vi "Teleop.vi"(10 "Match Info":T1={"Autonomous Elapsed Seconds"=0.0, "TeleOp Elapsed Seconds"=0.0, "Disabled Elapsed Seconds"=0.0, "Visited Autonomous"=FALSE, "Visited TeleOp"=FALSE, "Visited Disabled"=FALSE, "Autonomous Settings"={"Autonomous Style"=enum."Independent", "VI Refnum"=refnum}}, 11 "Call Context":T2) -> ()   [LabVIEW 2017]
doc: "This VI is called for each enabled TeleOp packet received from the DS. It is typically used to read from joysticks and other inputs and update I/O or setpoints for timed control loops. It should complete and return within 20 milliseconds or risk missing DS packets."
uses:
  <vilib>/Rock Robotics/WPI/DriverStation/WPI_DriverStationDerivedRobotMode.ctl
  <vilib>/Rock Robotics/WPI/DriverStation/WPI_DriverStationMatch Info.ctl
  <vilib>/Rock Robotics/WPI/Utilities/WPI_GetSetVariantRefNum.vi
  <vilib>/Rock Robotics/Network Tables/NT Write Boolean Array.vi
  <vilib>/Rock Robotics/Network Tables/NT Write Numeric Array.vi
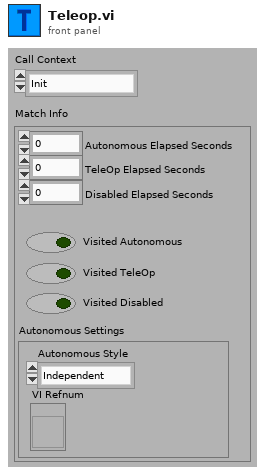
[diagram p1: front panel]
types:
  T1 = typedef "WPI_DriverStationMatch Info.ctl" = cluster{"Autonomous Elapsed Seconds":dbl, "TeleOp Elapsed Seconds":dbl, "Disabled Elapsed Seconds":dbl, "Visited Autonomous":bool, "Visited TeleOp":bool, "Visited Disabled":bool, "Autonomous Settings":cluster{"Autonomous Style":enum16{"Iterative", "Independent"}, "VI Refnum":refnum<vi>}}
  T2 = typedef "WPI_DriverStationDerivedRobotMode.ctl" = enum16{"Init", "Execute", "Stop"}
  T3 = typedef "WPI_JoystickDevRef.ctl" = cluster{"Device":T4}
  T4 = typedef "WPI_JoystickDeviceEnum.ctl" = enum16{"USB 0", "USB 1", "USB 2", "USB 3", "USB 4", "USB 5"}
  T5 = typedef "Command Status Info.ctl" = cluster{"Name":string, "Status":T6, "notifier out":T7}
  T6 = typedef "Completion Status.ctl" = enum16{"Successful", "Aborted", "Incomplete"}
  T7 = typedef "Completion Notifier.ctl" = refnum<notifier>
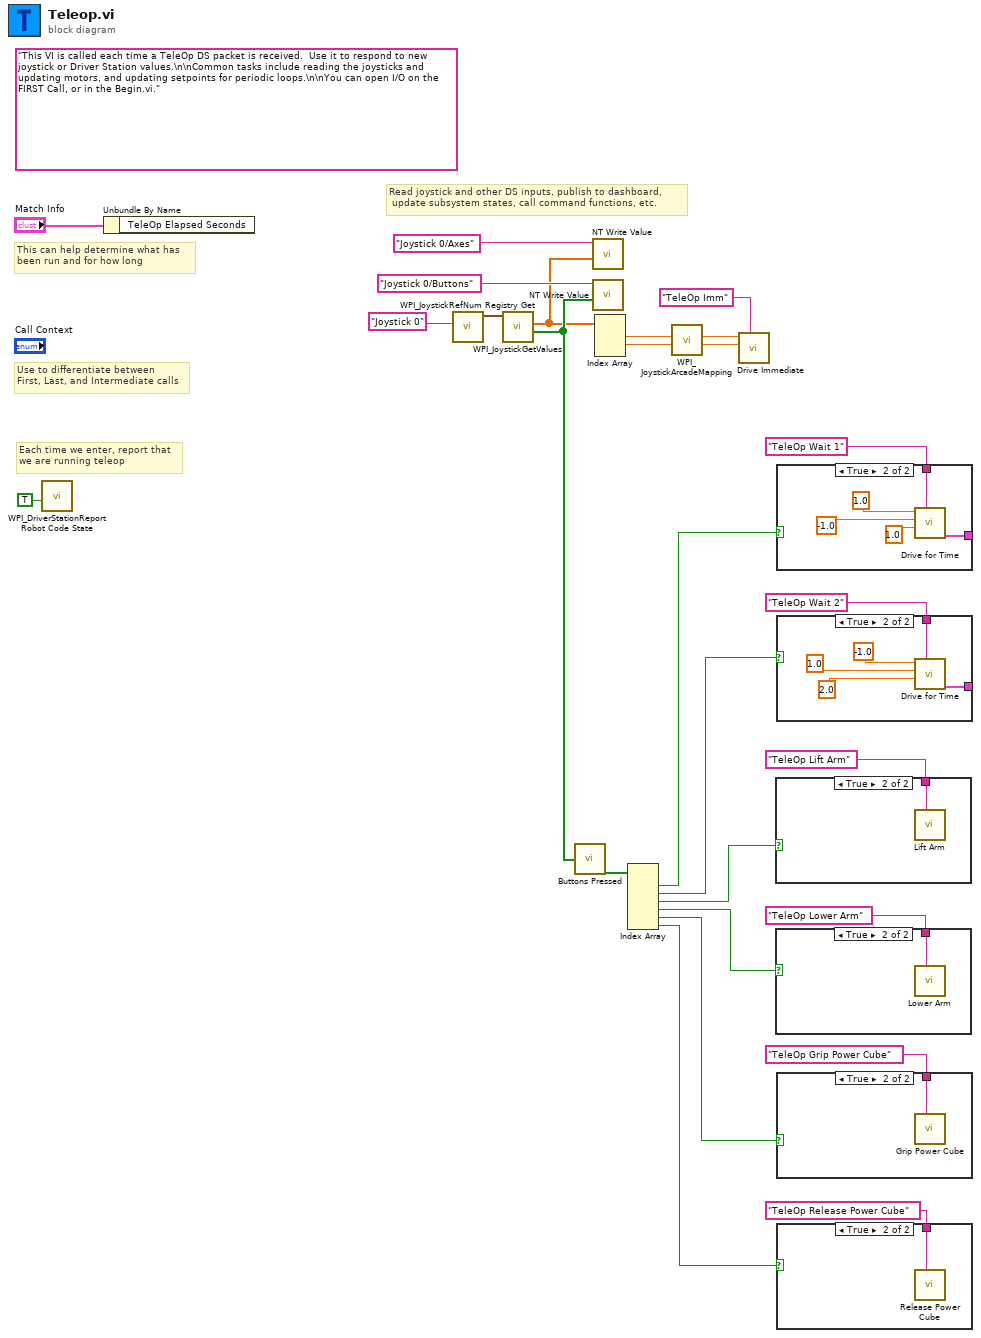
[diagram p0: block diagram]
diagram:
  (unwired) "This VI is called each time a TeleOp DS packet is received.  Use it to respond to new joystick or Driver Station values.\n\nCommon tasks include reading the joysticks and updating motors, and updating setpoints for periodic loops.\n\nYou can open I/O on the FIRST Call, or in the Begin.vi."
  # "Read joystick and other DS inputs, publish to dashboard,\n update subsystem states, call command functions, etc."
  # "Each time we enter, report that\nwe are running teleop"
  # "Use to differentiate between\nFirst, Last, and Intermediate calls"
  # "This can help determine what has\nbeen run and for how long"
  n1 = call <vilib>:"WPI_DriverStationReport Robot Code State.vi"("TeleOp"=TRUE ("Autonomous")) -> ()  [unwired: 10 in, 1 out]
  n2 = Unbundle By Name("Match Info") -> ()  [unwired: 1 out]
  n3 = call <vilib>:"WPI_JoystickRefNum Registry Get.vi"("refnum name"="Joystick 0") -> ("JoystickDevRef"=w23:T3)  [unwired: 1 in, 9 out]
  n4 = call <vilib>:"WPI_JoystickGetValues.vi"("JoystickDevRef"=w23) -> ("Buttons"=w11:bool[], "Axes"=w10:dbl[])  [unwired: 6 in, 3 out]
  n5 = call "Buttons Pressed.vi"("Button Values"=w11) -> ("Button Presses"=w19:bool[])
  n6 = call-poly <vilib>:"NT Write Value.vi"("Numeric Array"=w10, "Name"="Joystick 0/Axes") -> ()  [unwired: 9 in, 1 out]
  n7 = call-poly <vilib>:"NT Write Value.vi"("Boolean Array"=w11, "Name"="Joystick 0/Buttons") -> ()  [unwired: 9 in, 1 out]
  n8 = Index Array(array=w10) -> (element #1=w14:dbl, element #2=w13:dbl)  [unwired: 3 in, 1 out]
  n9 = Index Array(array=w19) -> (element #1=w18:bool, element #2=w17:bool, element #3=w4:bool, element #4=w3:bool, element #5=w2:bool, element #6=w1:bool)  [unwired: 6 in]
  n10 = call <vilib>:"WPI_JoystickArcadeMapping.vi"("Y axis value"=w13, "X axis value"=w14) -> ("Right Motor Value"=w15:dbl, "Left Motor Value"=w16:dbl)  [unwired: 8 in]
  n11 = call "Drive Immediate.vi"("Description"="TeleOp Imm", "Right Setpoint"=w15, "Left Setpoint"=w16) -> ()  [unwired: 8 in, 1 out]
  n12 = case shown="True" w4 {
    tunnel: "TeleOp Lift Arm" ("Description") -> [_ w27]
    frame False {
    }
    frame True {
      n13 = call "Lift Arm.vi"("Description"=w27) -> ()  [unwired: 10 in, 1 out]
    }
  }
  n14 = case shown="True" w3 {
    tunnel: "TeleOp Lower Arm" ("Description") -> [_ w28]
    frame False {
    }
    frame True {
      n15 = call "Lower Arm.vi"("Description"=w28) -> ()  [unwired: 10 in, 1 out]
    }
  }
  n16 = case shown="True" w18 {
    tunnel: [_ w32] -> _
    tunnel: "TeleOp Wait 1" ("Description") -> [_ w31]
    frame False {
    }
    frame True {
      n17 = call "Drive for Time.vi"("Description"=w31, "Seconds"=1.0, "Right Speed"=-1.0, "Left Speed"=1.0) -> ("Command Info Out"=w32:T5)  [unwired: 6 in, 1 out]
    }
  }
  n18 = case shown="True" w17 {
    tunnel: [_ w36] -> _
    tunnel: "TeleOp Wait 2" ("Description") -> [_ w35]
    frame False {
    }
    frame True {
      n19 = call "Drive for Time.vi"("Description"=w35, "Seconds"=2.0, "Right Speed"=1.0, "Left Speed"=-1.0) -> ("Command Info Out"=w36:T5)  [unwired: 6 in, 1 out]
    }
  }
  n20 = case shown="True" w2 {
    tunnel: "TeleOp Grip Power Cube" ("Description") -> [_ w39]
    frame False {
    }
    frame True {
      n21 = call "Grip Power Cube.vi"("Description"=w39) -> ()  [unwired: 10 in, 1 out]
    }
  }
  n22 = case shown="True" w1 {
    tunnel: "TeleOp Release Power Cube" ("Description") -> [_ w40]
    frame False {
    }
    frame True {
      n23 = call "Release Power Cube.vi"("Description"=w40) -> ()  [unwired: 10 in, 1 out]
    }
  }
